vi "Lectura y escritura de datos.vi"(5 "error in (no error)":errorcluster, 6 "Numeric in":dbl, 9 "append to file? (new file:F)":bool, 10 "Medición":string, 11 "Path":path) -> (1 "Numeric out":dbl, 2 "Array":dbl[](array[numeric]), 3 "Array 2":dbl[](array[numeric]))   [LabVIEW 2017]
uses:
  <vilib>/Utility/file.llb/Write Delimited Spreadsheet (DBL).vi
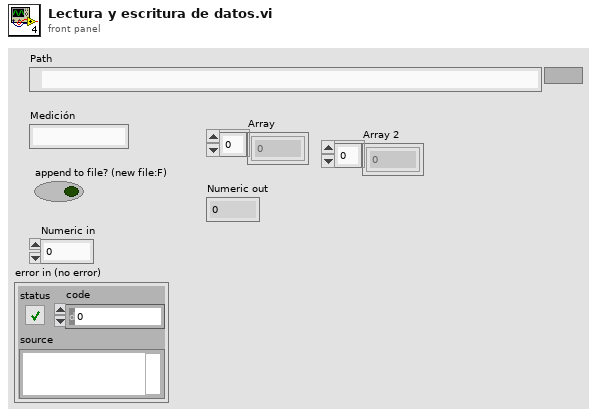
[diagram p1: front panel]
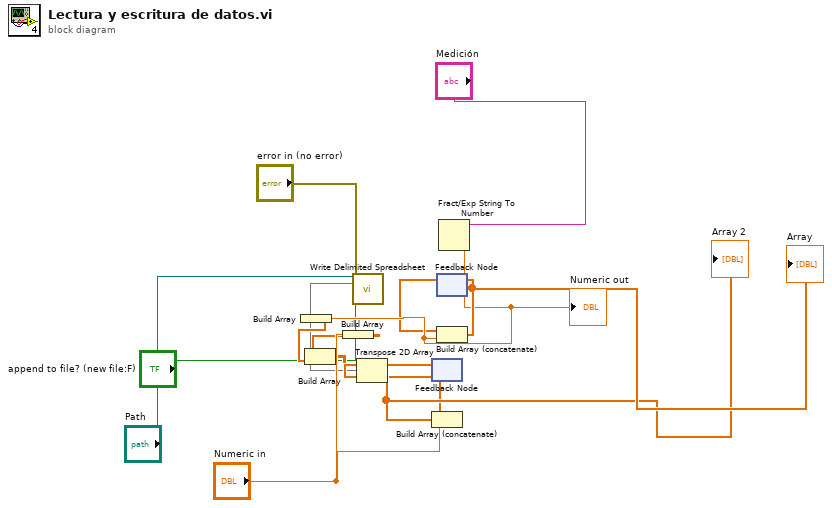
[diagram p0: block diagram]
diagram:
  n1 = Build Array("Numeric in") -> (w8:dbl[])
  n2 = feedback #1() -> (w11:dbl[])  [unwired: 1 in]
  n3 = Build Array (concatenate)(w11, "Numeric in") -> (w12:dbl[])
  "Array 2" <- w12
  n4 = feedback-in #1(w12) -> ()
  n5 = feedback #2() -> (w2:dbl[])  [unwired: 1 in]
  n6 = Fract/Exp String To Number(string="Medición") -> (number=w10:dbl)  [unwired: 3 in, 1 out]
  "Numeric out" <- w10
  n7 = Build Array(w10) -> (w9:dbl[])
  n8 = Build Array(w8, w9) -> (w6:dbl[][])
  n9 = Transpose 2D Array(2D array=w6) -> (transposed array=w7:dbl[][])
  n10 = call-poly <vilib>:"Write Delimited Spreadsheet.vi"("file path (dialog if empty)"="Path", "2D data"=w7, "append to file? (new file:F)"="append to file? (new file:F)", "error in (no error)"="error in (no error)") -> ()  [unwired: 10 in, 2 out]
  n11 = Build Array (concatenate)(w2, w10) -> (w13:dbl[])
  "Array" <- w13
  n12 = feedback-in #2(w13) -> ()
